vi "TempCtrlMonitor.vi"() -> ()   [LabVIEW 2015]
doc: "This is a control interface for using the digital temperature controller.\n\nThis interface is designed to be used in a stand-alone manner: a driver is also provided for low level, programmatic control and is used in the implementation of this GUI (see YbTempCtrl.lvlib)."
uses:
  Driver/Typedefs/OutputChannelTypedef.ctl
  Driver/Typedefs/InputChannelTypedef.ctl
  controls/ChannelSelection.ctl
  controls/ChannelSettings.ctl
  controls/UI Data.ctl
  controls/BridgeSettings.ctl
  <vilib>/Utility/error.llb/DialogType.ctl
  support/Message Queue/Enqueue Message (Single).vi
  support/Message Queue/Enqueue Message (Array).vi
  <vilib>/Utility/error.llb/Error Cluster From Error Code.vi
  <vilib>/ErrorRing/Error Ring.xnode
  support/Message Queue/Message Queue.lvlib
  support/User Event - Stop/User Event - Stop.lvlib
  Driver/YbTempCtrl.lvlib
panel:
  out "Data is logging":bool
  in  "Trigger time / s":i32=5 min=1
  in  "Tab Control":enum32{"Logging", "Control"}(tab)
  in  "Config input channel selector":T1
  in  "Input arm settings":T3(array[cluster])=[{"Enum string"="1T", "Enum ID"=0, "Input arm settings"={"Convert?"=FALSE, "Config"={"Vref"=1.25, "Rgain"=100000.0, "Rset"=10000.0, "Rseries"=1000.0, "Input polarity?"=FALSE}}}, {"Enum string"="2T", "Enum ID"=1, "Input arm settings"={"Convert?"=FALSE, "Config"={"Vref"=1.25, "Rgain"=100000.0, "Rset"=10000.0, "Rseries"=1000.0, "Input polarity?"=FALSE}}}, {"Enum string"="TMP", "Enum ID"=2, "Input arm settings"={"Convert?"=FALSE, "Config"={"Vref"=1.25, "Rgain"=100000.0, "Rset"=10000.0, "Rseries"=1000.0, "Input polarity?"=FALSE}}}, {"Enum string"="POW", "Enum ID"=3, "Input arm settings"={"Convert?"=FALSE, "Config"={"Vref"=1.25, "Rgain"=100000.0, "Rset"=10000.0, "Rseries"=1000.0, "Input polarity?"=FALSE}}}]
  in  "Output channel selection":T4=[{"Channel name"="1", "Enum id"=0, "Logging?"=FALSE}, {"Channel name"="2", "Enum id"=1, "Logging?"=FALSE}, {"Channel name"="3", "Enum id"=2, "Logging?"=FALSE}, {"Channel name"="4", "Enum id"=3, "Logging?"=FALSE}, {"Channel name"="BPA", "Enum id"=4, "Logging?"=FALSE}, {"Channel name"="BPB", "Enum id"=5, "Logging?"=FALSE}]
  in  "Input channel selection":T4=[{"Channel name"="1T", "Enum id"=0, "Logging?"=FALSE}, {"Channel name"="2T", "Enum id"=1, "Logging?"=FALSE}, {"Channel name"="TMP", "Enum id"=2, "Logging?"=FALSE}, {"Channel name"="POW", "Enum id"=3, "Logging?"=FALSE}]
  in  "Enable logging":bool
  in  "Log file prefix":string="Temperature log"
  in  "Log file directory":path
  in  "Reset":bool
  in  "VISA resource name":refnum<visa-resource-name>
  in  "Error alert group":enum32{"Page 1", "Page 2"}(tab)
  in  "Error abort":bool
  in  "Error ignore":bool
  out "Reported Error":string="20:32:20.341 21/11/2016 - Code -1073807346: 'VISA Open in YbTempCtrl.lvlib:Initialize.vi->TempCtrlMonitor.vi'"
  out "Output error":errorcluster={"status"=TRUE, "code"=-1073807346, "source"="VISA Write in YbTempCtrl.lvlib:Query-ControlSignal.vi->TempCtrlMonitor.vi"}
  out "Input error":errorcluster={"status"=TRUE, "code"=9999, "source"="Error from device: \"\""}
  out "Reading":dbl(graph)=nan
  in  "Input channel":T1
  in  "Output channel":T5
  in  "Start Lock":bool caption="Start Lock Outer"
  in  "Start Const.Voltage":bool caption="Start Lock Outer"
  in  "CtrlVoltage":dbl=nan caption="Output voltage / V"
  in  "Min_Ctrl":dbl caption="Minimum / V"
  in  "Max_Ctrl":dbl caption="Maximum / V"
  in  "Lock settings":T6={"K / V/V"=0.0, "T_I / s"=0.0, "T_D / s"=0.0, "Target Error / C"=0.0, "N"=10.0}
  in  "Exit":bool
  # "Log file setup"
  # "VISA config"
  # "Select which channels should be logged here. These will \nbe written to the log file regardless of which channel is \ndisplayed in the \"Control\" tab as long as \"Enable logging\" \nis set."
  # "Thermistor config"
  # "Enter the settings associated with a particular channel\nhere and then select \"Convert?\" in order to convert \nvoltages to temperatures on display\nN.B. Log files always contain raw voltages"
  # "Log files will be created with the current date and time appended to the prefix given here"
  # "Error reported:"
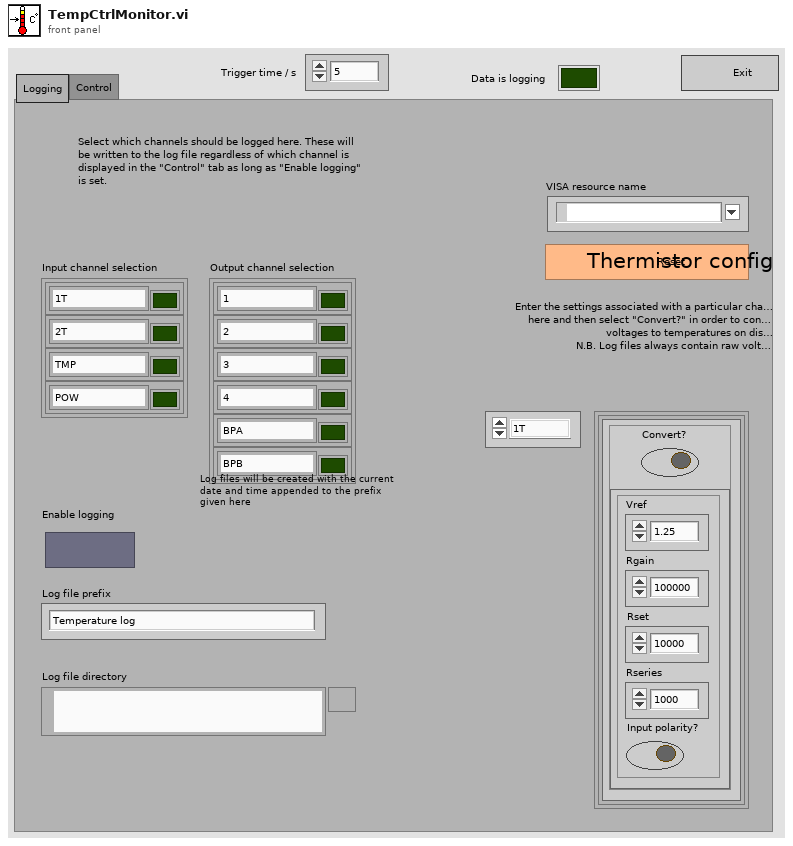
[diagram p1: front panel]
types:
  T1 = typedef "YbTempCtrl.lvlib/InputChannelTypedef.ctl" = enum16{"1T", "2T", "TMP", "POW"}
  T2 = typedef "ChannelSettings.ctl" = cluster{"Convert?":bool, "Config":cluster{"Vref":dbl, "Rgain":dbl, "Rset":dbl, "Rseries":dbl, "Input polarity?":bool}}
  T3 = cluster{"Enum string":string, "Enum ID":i16, "Input arm settings":T2}[]
  T4 = typedef "ChannelSelection.ctl" = cluster{"Channel name":string, "Enum id":u16, "Logging?":bool}[]
  T5 = typedef "YbTempCtrl.lvlib/OutputChannelTypedef.ctl" = enum16{"1", "2", "3", "4", "BPA", "BPB"}
  T6 = cluster{"K / V/V":dbl, "T_I / s":dbl, "T_D / s":dbl, "Target Error / C":dbl, "N":dbl}
  T7 = typedef "UI Data.ctl" = cluster{"VISA resource name":refnum<visa-resource-name>, "Log dir":refnum<vi>, "Log file":refnum<file>, "Outer PID State":string, "Inner PID State":string, "MAX_VOLTAGE":dbl, "Channel 1 bridge settings":T8, "Channel 2 bridge settings":T8, "Current Levels":cluster{"Control 1":dbl, "Control 2":dbl, "Control BP":dbl, "Error 1t":dbl, "Error 1v":dbl, "Error 2t":dbl, "Error 2v":dbl}, "Data is logging":refnum<vi>, "Output channel ref":refnum<vi>, "Output channel selection ref":refnum<vi>, "Input channel ref":refnum<vi>, "Input channel selection ref":refnum<vi>, "Log data?":bool, "Error reported?":bool, "Input arm settings":cluster{"Enum string":string, "Enum ID":i16, "Input arm settings":T2}[], "Input arm settings ref":refnum<vi>}
  T8 = typedef "BridgeSettings.ctl" = cluster{"Rgain":dbl, "Rset":dbl, "Vref":dbl, "Input polarity?":bool, "Rtherm_25":dbl}
  T9 = typedef "Message Queue.lvlib/All Message Queues.ctl" = cluster{"UI":refnum<queue>}
  T10 = enum8{"Enabled", "Disabled", "Disabled and Grayed Out"}
  T11 = typedef "YbTempCtrl.lvlib/OutputChannelTypedef.ctl" = enum16{"1", "2", "BP"}
  T12 = cluster{"K":dbl, "T_I / s":dbl, "T_D / s":dbl, "Target Error / V":dbl, "N":dbl}
  T13 = cluster{"Lock settings":cluster{"K":dbl, "T_I / s":dbl, "T_D / s":dbl, "Target Error / C":dbl, "N":dbl}, "Output channel":T5, "Input channel":T1}
  T14 = cluster{"Output channel":T5, "Max_Ctrl1":dbl, "Min_Ctrl1":dbl}
  T15 = cluster{"Output channel":T5, "Voltage outer":dbl}
  T16 = typedef "DialogType.ctl" = u16
  T17 = cluster{"seconds since 1Jan1904":timestamp, dbl[]}
  T18 = cluster{"K":dbl, "T_I / s":dbl, "T_D / s":dbl, "Target Error / C":dbl, "N":dbl}
  T19 = cluster{"Enum string":string, "Enum ID":i16, "Input arm settings":T2}
  T20 = cluster{"Vref":dbl, "Rgain":dbl, "Rset":dbl, "Rseries":dbl, "Input polarity?":bool}
  T21 = cluster{"Lock settings":cluster{"K / V/V":dbl, "T_I / s":dbl, "T_D / s":dbl, "Target Error / C":dbl, "N":dbl}, "Output channel":T5, "Input channel":T1}
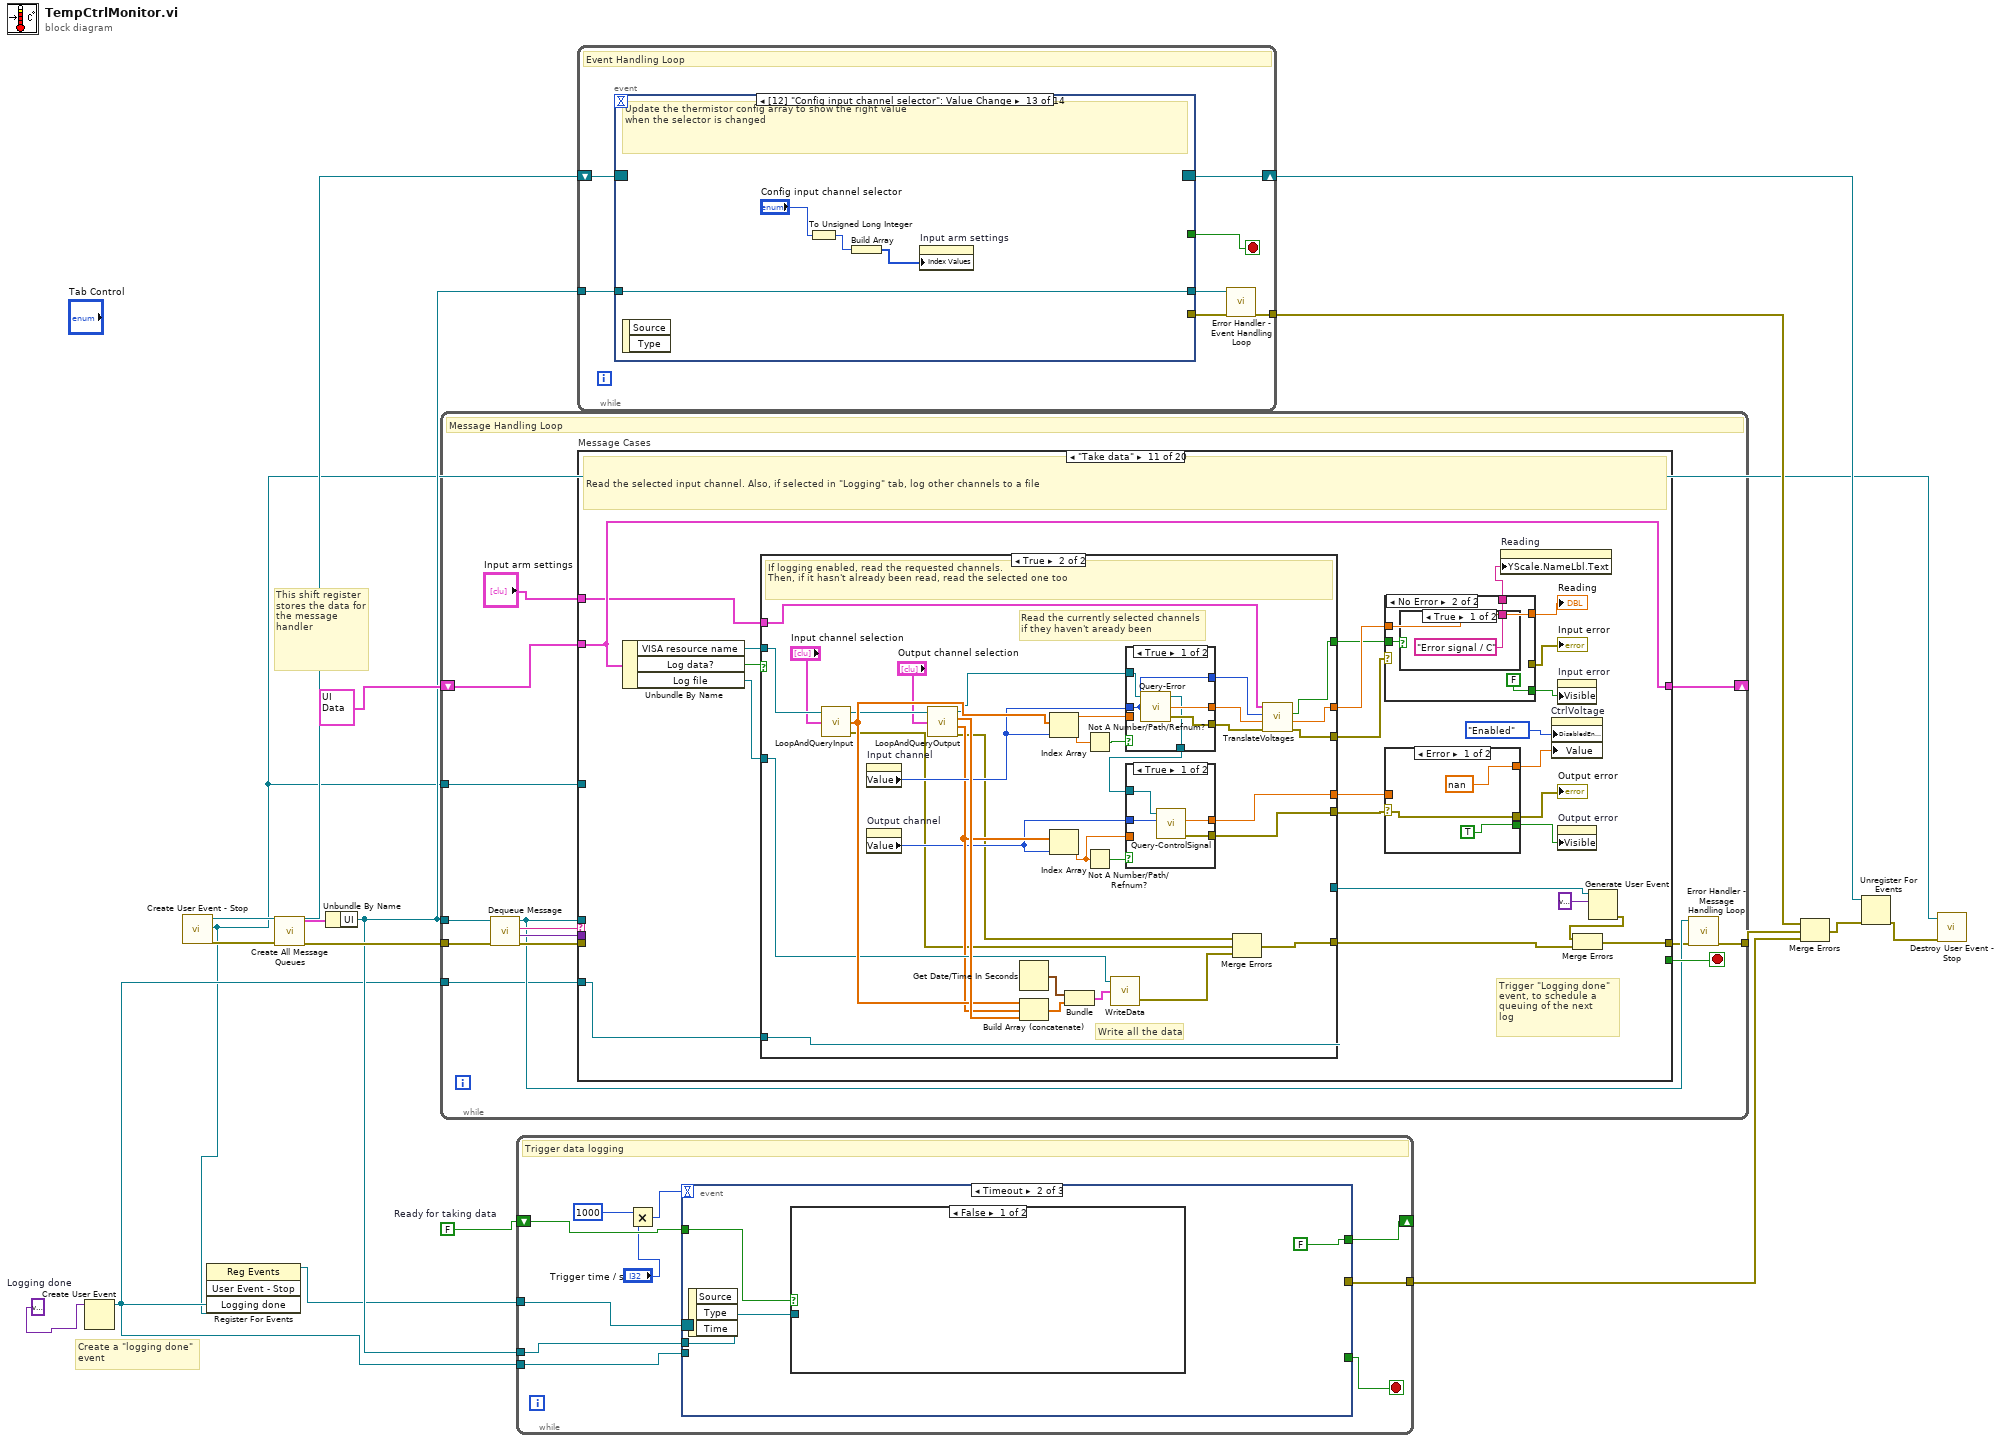
[diagram p0: block diagram]
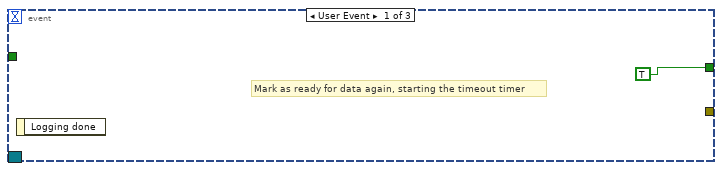
[diagram p2: hidden frame]
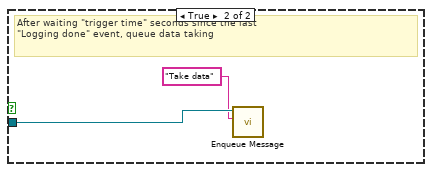
[diagram p3: hidden frame]
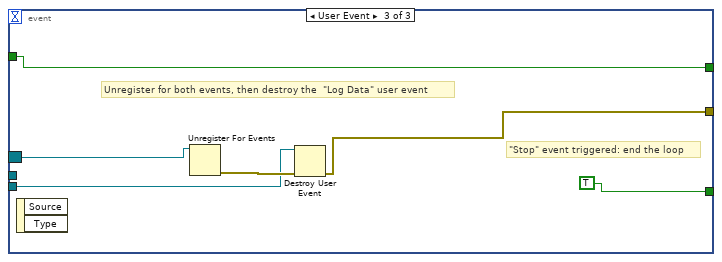
[diagram p4: hidden frame]
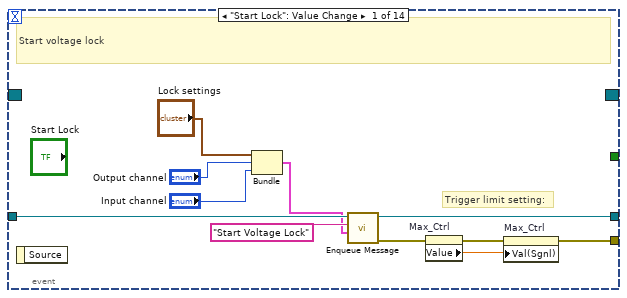
[diagram p5: hidden frame]
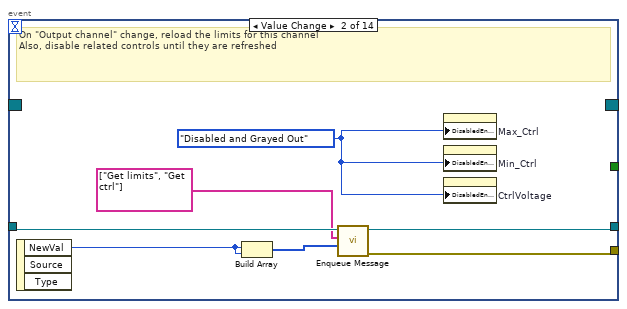
[diagram p6: hidden frame]
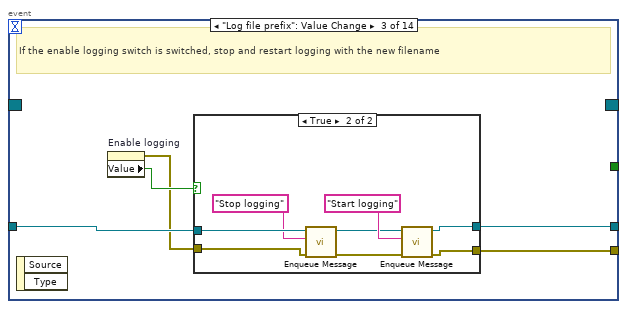
[diagram p7: hidden frame]
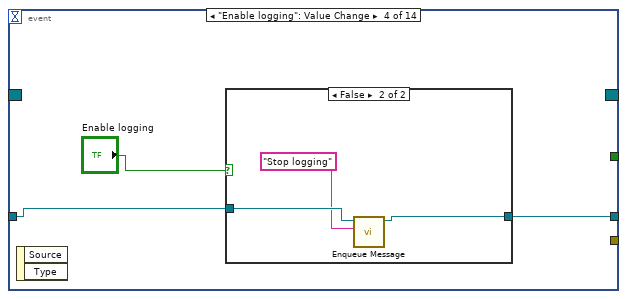
[diagram p9: hidden frame]
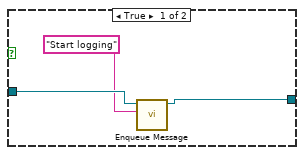
[diagram p10: hidden frame]
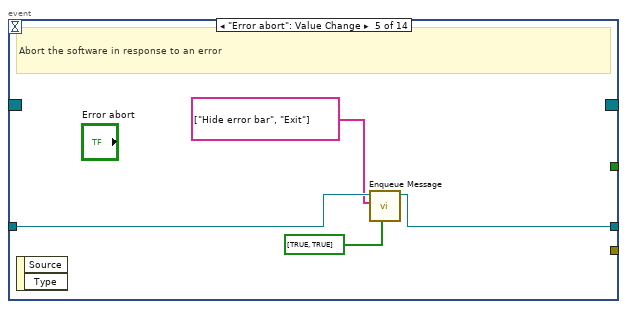
[diagram p11: hidden frame]
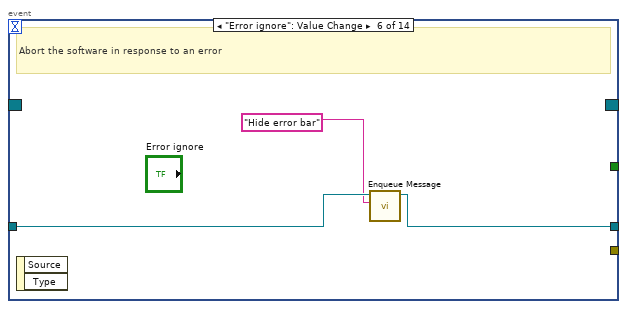
[diagram p12: hidden frame]
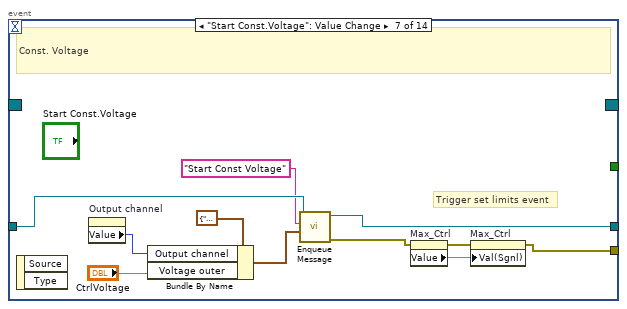
[diagram p13: hidden frame]
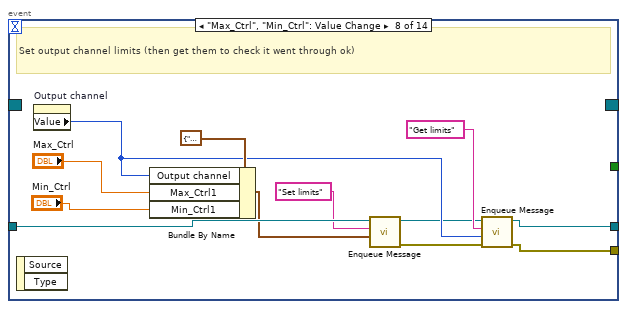
[diagram p14: hidden frame]
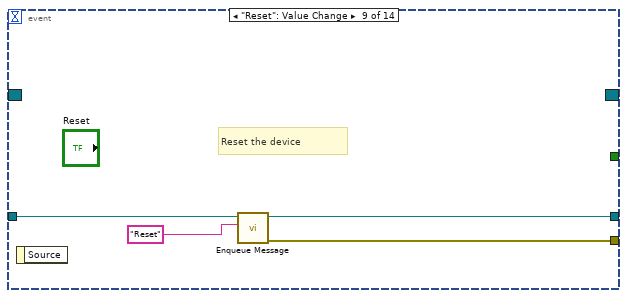
[diagram p15: hidden frame]
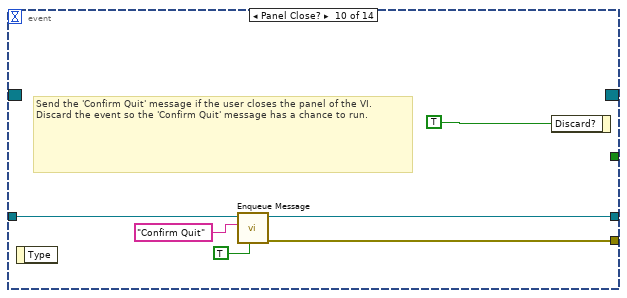
[diagram p16: hidden frame]
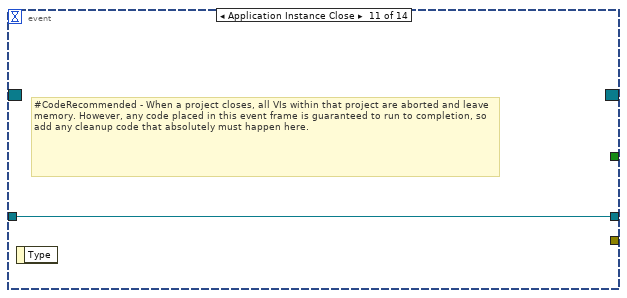
[diagram p17: hidden frame]
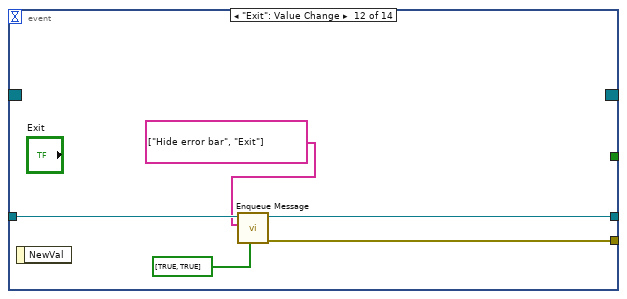
[diagram p18: hidden frame]
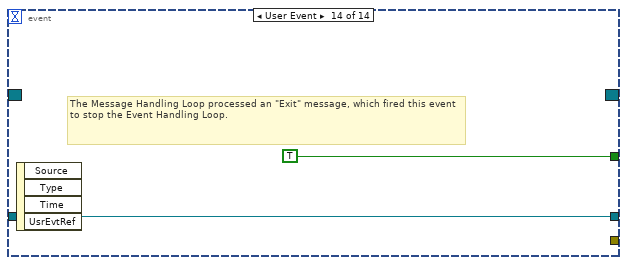
[diagram p19: hidden frame]
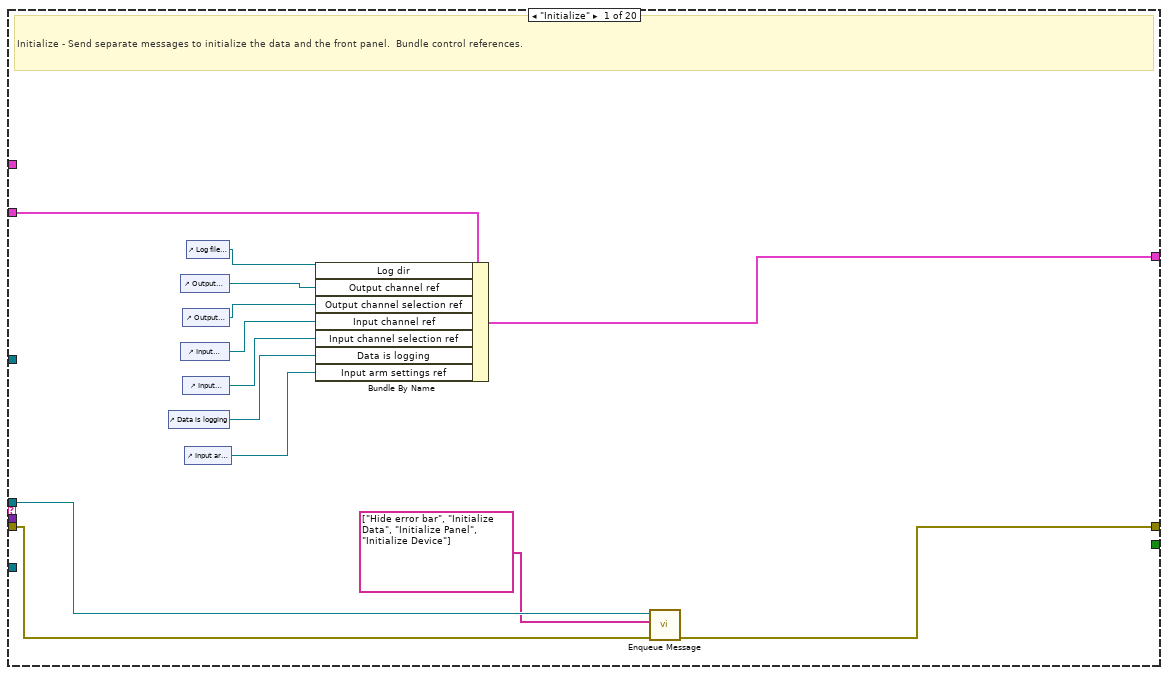
[diagram p20: hidden frame]
diagram:
  w1 = FALSE  # Ready for taking data
  w8 = variant  # Logging done
  # "Create a \"logging done\"\nevent"
  # "This shift register stores the data for the message handler"
  n1 = Create User Event(user event datatype=w8) -> (user event=w4:refnum<user-event>)  [unwired: 1 in, 1 out]
  n2 = call "Create User Event - Stop.vi"() -> ("error out"=w15:errorcluster, "User Event - Stop"=w3:refnum<user-event>, "Stop Event Registration Refnum"=w9:refnum<event-registration>)  [unwired: 9 in]
  n3 = register-events(w3, w4) -> (reference out=w2:refnum<event-registration>)  [unwired: 2 in, 1 out]
  n4 = call "Create All Message Queues.vi"("error in (no error)"=w15) -> ("error out"=w17:errorcluster, "Message Queues out"=w16:T9)  [unwired: 9 in]
  n5 = Unbundle By Name(w16) -> ("UI"=w10:refnum<queue>)
  n6 = while {
    tunnel: w10 -> [w23]
    shift-right: [w30] -> _
    shift-left: T7 {"VISA resource name"="", "Log dir"=refnum, "Log file"=refnum, "Outer PID State"="", "Inner PID State"="", "MAX_VOLTAGE"=0.0, "Channel 1 bridge settings"={"Rgain"=0.0, "Rset"=0.0, "Vref"=0.0, "Input polarity?"=FALSE, "Rtherm_25"=0.0}, "Channel 2 bridge settings"={"Rgain"=0.0, "Rset"=0.0, "Vref"=0.0, "Input polarity?"=FALSE, "Rtherm_25"=0.0}, "Current Levels"={"Control 1"=0.0, "Control 2"=0.0, "Control BP"=0.0, "Error 1t"=0.0, "Error 1v"=0.0, "Error 2t"=0.0, "Error 2v"=0.0}, "Data is logging"=refnum, "Output channel ref"=refnum, "Output channel selection ref"=refnum, "Input channel ref"=refnum, "Input channel selection ref"=refnum, "Log data?"=FALSE, "Error reported?"=FALSE, "Input arm settings"=[], "Input arm settings ref"=refnum} ("Data Cluster") -> [w31]
    tunnel: w3 -> [w28]
    tunnel: w17 -> [w27]
    tunnel: [w21] -> w7
    tunnel: w4 -> [w19]
    stop <- w29 stop-if-true
    # "Message Handling Loop"
    n7 = call "Dequeue Message.vi"("error in (no error)"=w27, "Message Queue"=w23) -> ("error out"=w26:errorcluster, "Message Data"=w24:variant, "Message"=w25:string, "dup Message Queue"=w22:refnum<queue>)  [unwired: 6 in]
    n8 = case "Message Cases" shown="\"Take data\"" w25 {
      selector: w25 -> [_ _ _ _ _ _ _ _ _ _ _ _ _ _ _ _ _ _ _ w399]
      tunnel: w22 -> [w42 _ w58 w89 _ w143 _ _ _ w174 _ _ w324 w337 _ _ _ _ w398 _]
      tunnel: w26 -> [w43 w55 w60 _ w121 w147 w150 w155 w164 w177 _ w286 w325 w339 _ _ _ _ w395 _]
      tunnel: [w44 w52 w63 w108 w119 w145 w148 w154 w165 w173 w204 w289 w322 w341 w342 w356 w374 w386 w396 w400] -> w20
      tunnel: w31 -> [w41 w54 w62 w104 w117 w146 w149 w153 w159 w170 w187 w288 w302 w340 w348 w364 w376 w384 w393 w401]
      tunnel: [w40 w53 w62 w103 w116 w146 w149 w152 w158 w179 w187 w288 w302 w340 w348 w364 w376 w384 w393 w401] -> w30
      tunnel: [_ _ _ _ _ _ _ _ _ _ _ _ _ _ _ _ _ _ TRUE _] -> w29
      tunnel: w24 -> [_ _ _ _ w120 _ _ _ _ _ _ _ w327 _ w349 w365 w377 w385 _ _]
      tunnel: w28 -> [_ _ _ _ _ _ _ _ _ _ _ _ _ _ _ _ _ _ w394 _]
      tunnel: w19 -> [_ _ _ _ _ _ _ _ _ _ w207 _ _ _ _ _ _ _ _ _]
      tunnel: "Input arm settings" -> [_ _ _ _ _ _ _ _ _ _ w186 _ w308 _ _ _ _ _ _ _]
      frame "Initialize" {
        # "Initialize - Send separate messages to initialize the data and the front panel.  Bundle control references."
        n9 = control-ref of="Data is logging"() -> (w33:refnum<vi>)
        n10 = control-ref of="Output channel"() -> (w37:refnum<vi>)
        n11 = control-ref of="Input channel"() -> (w36:refnum<vi>)
        n12 = control-ref of="Output channel selection"() -> (w34:refnum<vi>)
        n13 = control-ref of="Input channel selection"() -> (w35:refnum<vi>)
        n14 = control-ref of="Input arm settings"() -> (w32:refnum<vi>)
        n15 = control-ref of="Log file directory"() -> (w39:refnum<vi>)
        n16 = Bundle By Name(cluster=w41, "Log dir"=w39, "Output channel ref"=w37, "Output channel selection ref"=w34, "Input channel ref"=w36, "Input channel selection ref"=w35, "Data is logging"=w33, "Input arm settings ref"=w32) -> (w40:T7)
        n17 = call-poly "Enqueue Message.vi"("error in (no error)"=w43, "Message Array"=string[] ["Hide error bar", "Initialize Data", "Initialize Panel", "Initialize Device"], "Message Queue"=w42) -> ("error out"=w44:errorcluster)  [unwired: 7 in, 1 out]
      }
      frame "Initialize Data" {
        w45 = nan
        w51 = "?"
        # "Initialize Data - Initialize the state data cluster."
        n18 = Bundle(w45, w45, w45, w45, w45, w45, w45) -> (w46:cluster{dbl, dbl, dbl, dbl, dbl, dbl, dbl})  [unwired: 1 in]
        n19 = Bundle By Name(cluster=w54, "VISA resource name"="VISA resource name", "Outer PID State"=w51, "Inner PID State"=w51, "MAX_VOLTAGE"=15.0, "Channel 1 bridge settings"=T8 {"Rgain"=42000.0, "Rset"=9500.0, "Vref"=1.0, "Input polarity?"=FALSE, "Rtherm_25"=10000.0}, "Channel 2 bridge settings"=T8 {"Rgain"=42000.0, "Rset"=9500.0, "Vref"=1.0, "Input polarity?"=FALSE, "Rtherm_25"=10000.0} ("Channel 1 bridge settings"), "Current Levels"=w46) -> (w53:T7)
        n20 = Merge Errors(w55) -> (w52:errorcluster)
      }
      frame "Initialize Device" {
        # "No reset"
        # "Initialize Device - Start comms with the PID controller"
        n21 = Unbundle By Name(w62) -> ("VISA resource name"=w56:refnum<visa-resource-name>)
        n22 = call "Initialize.vi"("error in (no error)"=w60, "Reset (True)"=FALSE, "VISA resource name"=w56) -> ("error out"=w59:errorcluster)  [unwired: 7 in, 1 out]
        n23 = case shown="Error" w59 {
          selector: w59 -> [w64 w76]
          tunnel: w58 -> [_ w72]
          tunnel: [w64 w69] -> w57
          tunnel: w56 -> [_ w65]
          frame No Error {
            # "No error"
          }
          frame Error {
            w75 = T16 0 items=["no dialog", "OK message", "continue or stop message", "OK message + warnings", "continue/stop + warnings"] ("type of dialog (OK msg:1)")
            # "Error initialising the device. Abort execution since there's\nno point continuing. (This code is here to override the default\nerror handler which would just pop up an error bar)"
            n24 = call <vilib>:"Simple Error Handler.vi"("type of dialog (OK msg:1)"=w75, "error in (no error)"=w76) -> ("code out"=w66:i32, "source out"=w67:string)  [unwired: 3 in, 3 out]
            n25 = Format Into String(format string="An error occured in device initialisation.\nCOM port: \"%s\"\nError code: %d\nError message: \"%s\"", w65, w66, w67) -> (resulting string=w73:string)  [unwired: 2 in, 1 out]
            n26 = One Button Dialog(message=w73, button name ("OK")="Abort...") -> ()  [unwired: 1 out]
            n27 = call-poly "Enqueue Message.vi"("Priority Message? (F)"=TRUE, "Message"="Exit", "Message Queue"=w72) -> ("error out"=w69:errorcluster)  [unwired: 7 in, 1 out]
          }
        }
        n28 = Merge Errors(w57) -> (w63:errorcluster)
      }
      frame "Initialize Panel" {
        w95 = FALSE
        # "Trigger the index changed event"
        # "Trigger taking of first data\nFrom here on, \"Take data\" will retrigger itself"
        # "Trigger reloading of limits"
        # "Set logging indicators to false (they will be updated later)"
        # "Initialize Panel - Initialize the appearance of the front panel here."
        n29 = Unbundle By Name(w104) -> ("Data is logging"=w107:refnum<vi>, "Output channel ref"=w106:refnum<vi>, "Output channel selection ref"=w105:refnum<vi>, "Input channel ref"=w102:refnum<vi>, "Input channel selection ref"=w101:refnum<vi>, "Input channel ref"=w88:refnum<vi>, "Input arm settings ref"=w82:refnum<vi>)
        n30 = property on="Output channel" class="Enum (strict)"() -> ("Value"=w99:T5)  [unwired: 2 in, 2 out]
        n31 = call-poly "Enqueue Message.vi"("Message Data"=w99, "Message"="Get limits", "Message Queue"=w89) -> ("error out"=w94:errorcluster, "dup Message Queue"=w93:refnum<queue>)  [unwired: 7 in]
        n32 = property on="Enable logging" class="Bool (strict)"() -> ("Value"=w96:bool)  [unwired: 2 in, 2 out]
        n33 = property class="Bool (strict)"(reference=w107, "Value"=w95) -> (error out=w86:errorcluster)  [unwired: 1 in, 1 out]
        n34 = Bundle By Name(cluster=w104, "Log data?"=w95) -> (w103:T7)
        n35 = case shown="True" w96 {
          tunnel: w94 -> [w110 w115]
          tunnel: w93 -> [w109 w114]
          tunnel: "Start logging" ("Message") -> [_ w113]
          tunnel: [w110 w112] -> w91
          tunnel: [w109 w111] -> w90
          frame False {
          }
          frame True {
            n36 = call-poly "Enqueue Message.vi"("error in (no error)"=w115, "Message"=w113, "Message Queue"=w114) -> ("error out"=w112:errorcluster, "dup Message Queue"=w111:refnum<queue>)  [unwired: 7 in]
          }
        }
        n37 = control-ref of="Config input channel selector"() -> (w77:refnum<vi>)
        n38 = call "PopulateChannelArray.vi"("Channel Selection ref"=w105, "Enum in"=w106) -> ("error out"=w85:errorcluster)  [unwired: 2 in]
        n39 = call "PopulateChannelArray.vi"("Channel Selection ref"=w101, "Enum in"=w102) -> ("error out"=w84:errorcluster)  [unwired: 2 in]
        n40 = call "PopulateChannelSettingsArray.vi"("Update size?"=FALSE, "Input arm settings ref"=w82, "Enum in"=w88) -> ("error out"=w81:errorcluster)  [unwired: 1 in]
        n41 = property class="Enum (strict)"(reference=w77, error in=w81) -> (reference out=w78:refnum<vi>, error out=w79:errorcluster, "Value"=w80:T1)
        n42 = call-poly "Enqueue Message.vi"("error in (no error)"=w91, "Message"="Take data", "Message Queue"=w90) -> ("error out"=w92:errorcluster)  [unwired: 7 in, 1 out]
        n43 = property class="Enum (strict)"(reference=w78, error in=w79, "Val(Sgnl)"=w80) -> (error out=w83:errorcluster)  [unwired: 1 out]
        n44 = Merge Errors(w86, w85, w84, w83, w92) -> (w108:errorcluster)
      }
      frame "Error" {
        # "#CodeRecommended - If you ever change the name of this \"Error\" message, you'll need to update the name in the Check Loop Error.vi as well."
        # "Error - Check the error message data and respond accordingly. This message is sent by the \"Error Handler\" VIs at the end of each loop in this application.\n\nResponse: show the error alert box, allowing the user to abort the program"
        n45 = Unbundle By Name(w117) -> ("Error reported?"=w118:bool)
        n46 = case shown="False" w118 {
          tunnel: w121 -> [w138 w140]
          tunnel: w120 -> [w137 _]
          tunnel: [w128 w140] -> w119
          tunnel: w117 -> [w124 w139]
          tunnel: [w123 w139] -> w116
          frame False {
            w134 = T16 0 items=["no dialog", "OK message", "continue or stop message", "OK message + warnings", "continue/stop + warnings"] ("type of dialog (OK msg:1)")
            # "Show the error bar"
            # "The error bar is not yet visible. Populate it with details of the error then show it"
            n47 = Variant To Data(error in=w138, type=errorcluster {"status"=FALSE, "code"=0, "source"=""} ("error constant"), Variant=w137) -> (data=w135:errorcluster, error out=w131:errorcluster)
            n48 = Get Date/Time In Seconds() -> (seconds since 1Jan1904=w125:timestamp)
            n49 = call <vilib>:"Simple Error Handler.vi"("type of dialog (OK msg:1)"=w134, "error in (no error)"=w135) -> ("code out"=w126:i32, "source out"=w127:string)  [unwired: 3 in, 3 out]
            n50 = Format Into String(format string="%T - Code %d: '%s'", error in=w131, w125, w126, w127) -> (resulting string=→"Reported Error":string, error out=w129:errorcluster)  [unwired: 1 in]
            n51 = Bundle By Name(cluster=w124, "Error reported?"=TRUE) -> (w123:T7)
            n52 = property on="Error alert group" class="TabCtl (strict)"(error in=w129, "Visible"=TRUE) -> (error out=w128:errorcluster)  [unwired: 1 in, 1 out]
          }
          frame True {
            # "An error is already visible. Leave it, since it's probably more useful than newer errors"
          }
        }
      }
      frame "Confirm Quit" {
        # "#CodeNeeded - If you want to provide an \"Are you sure\" dialog (or some other notification) before the application exits, place that code here. This message is typically sent from a Panel Close? event."
        # "Confirm Quit - Message that can confirm whether or not the user wants to exit the application."
        n53 = call-poly "Enqueue Message.vi"("Priority Message? (F)"=TRUE, "error in (no error)"=w147, "Message"="Exit", "Message Queue"=w143) -> ("error out"=w144:errorcluster)  [unwired: 6 in, 1 out]
        n54 = Merge Errors(w144) -> (w145:errorcluster)
      }
      frame "---Copy This Frame---" {
        # "Duplicate this frame when creating new messages.  Change this comment in the duplicated frame to describe this message."
        n55 = Merge Errors(w150) -> (w148:errorcluster)
      }
      frame "Hide error bar" {
        # "Hide the error bar"
        n56 = Bundle By Name(cluster=w153, "Error reported?"=FALSE) -> (w152:T7)
        n57 = property on="Error alert group" class="TabCtl (strict)"(error in=w155, "Visible"=FALSE) -> (error out=w154:errorcluster)  [unwired: 1 in, 1 out]
      }
      frame "Stop logging" {
        # "Mark logging as disabed: the event will not get re-triggered so logging will stop"
        n58 = Unbundle By Name(w159) -> ("Log file"=w162:refnum<file>)
        n59 = Not A Number/Path/Refnum?(number/path/refnum=w162) -> (NaN/Path/Refnum?=w161:bool)
        n60 = case shown="False" w161 {
          tunnel: w164 -> [w168 w169]
          tunnel: [w167 w169] -> w163
          tunnel: w162 -> [w166 _]
          frame False {
            n61 = Close File(refnum=w166, error in=w168) -> (error out=w167:errorcluster)  [unwired: 1 out]
          }
          frame True {
          }
        }
        n62 = Bundle By Name(cluster=w159, "Log data?"=FALSE, "Log file"=refnum<k0> refnum) -> (w158:T7)
        n63 = Merge Errors(w163) -> (w165:errorcluster)
      }
      frame "Start logging" {
        # "Open files for data logging with the given headers"
        n64 = call "GenFilenames.vi"("Controller name"="Log file prefix", "Default dir"="Log file directory") -> ("Log file"=w180:path)  [unwired: 1 in]
        n65 = call "GenerateHeaders.vi"("UI Data"=w170) -> ("Output headers"=w171:string)  [unwired: 1 in]
        n66 = call "OpenFile.vi"("error in (no error)"=w177, "Filepath"=w180, "Extra headers"=w171) -> ("error out"=w176:errorcluster, "File handle"=w178:refnum<file>)
        n67 = case shown="Error" w176 {
          selector: w176 -> [w182 w184]
          tunnel: [TRUE ("Data is logging") FALSE ("Data is logging")] -> w172
          tunnel: w174 -> [_ _]
          tunnel: [w182 _] -> w173
          frame No Error {
            # "Mark logging as enabled"
          }
          frame Error {
            # "Opening files failed! Report error"
            n68 = call <vilib>:"Simple Error Handler.vi"("error in (no error)"=w184) -> ()  [unwired: 4 in, 5 out]
          }
        }
        "Data is logging" <- w172
        n69 = Bundle By Name(cluster=w170, "Log file"=w178, "Log data?"=w172) -> (w179:T7)
        n70 = property on="Enable logging" class="Bool (strict)"("Value"=w172) -> ()  [unwired: 2 in, 2 out]
      }
      frame "Take data" {
        # "Trigger \"Logging done\"\nevent, to schedule a\nqueuing of the next\nlog"
        # "Read the selected input channel. Also, if selected in \"Logging\" tab, log other channels to a file"
        n71 = Unbundle By Name(w187) -> ("VISA resource name"=w209:refnum<visa-resource-name>, "Log data?"=w208:bool, "Log file"=w200:refnum<file>)
        n72 = case shown="True" w208 {
          tunnel: w209 -> [w237 w271]
          tunnel: [_ w266] -> w202
          tunnel: w207 -> [w238 w261]
          tunnel: [w228 w243] -> w196
          tunnel: [w238 w261] -> w205
          tunnel: [w232 w244] -> w201
          tunnel: w200 -> [_ w257]
          tunnel: [w234 w248] -> w193
          tunnel: [w233 w252] -> w192
          tunnel: [w227 w242] -> w191
          tunnel: w186 -> [w226 w241]
          frame False {
            # "If logging disabled, just read the currently selected channels"
            n73 = property on="Input channel" class="Enum (strict)"() -> ("Value"=w229:T1)  [unwired: 2 in, 2 out]
            n74 = property on="Output channel" class="Enum (strict)"() -> ("Value"=w236:T5)  [unwired: 2 in, 2 out]
            n75 = call "Query-Error.vi"("Input channel"=w229, "VISA resource name"=w237) -> ("error out"=w231:errorcluster, "Error Signal / V"=w230:dbl, "VISA resource name out"=w235:refnum<visa-resource-name>)  [unwired: 1 in]
            n76 = call "Query-ControlSignal.vi"("Output channel"=w236, "VISA resource name"=w235) -> ("error out"=w234:errorcluster, "Recalled Control signal / V"=w233:dbl)  [unwired: 7 in, 1 out]
            n77 = call "TranslateVoltages.vi"("Input arm settings"=w226, "Input channel"=w229, "Reading / V"=w230, "error in (no error)"=w231) -> ("Output is temperature?"=w227:bool, "Output"=w228:dbl, "error out"=w232:errorcluster)  [unwired: 1 in, 2 out]
          }
          frame True {
            # "Read the currently selected channels\nif they haven't aready been"
            # "Write all the data"
            # "If logging enabled, read the requested channels. \nThen, if it hasn't already been read, read the selected one too"
            n78 = call "LoopAndQueryInput.vi"("Input channel selection"="Input channel selection", "VISA Refnum in"=w271) -> ("error out"=w239:errorcluster, "Error signal / V"=w265:dbl[], "VISA resource name out"=w260:refnum<visa-resource-name>)  [unwired: 1 in]
            n79 = property on="Input channel" class="Enum (strict)"() -> ("Value"=w263:T1)  [unwired: 2 in, 2 out]
            n80 = property on="Output channel" class="Enum (strict)"() -> ("Value"=w250:T5)  [unwired: 2 in, 2 out]
            n81 = call "LoopAndQueryOutput.vi"("VISA Refnum in"=w260, "Output channel selection"="Output channel selection") -> ("VISA resource name out"=w256:refnum<visa-resource-name>, "Setpoint / V"=w270:dbl[], "Control signal / V"=w253:dbl[], "error out"=w240:errorcluster)  [unwired: 1 in]
            n82 = Get Date/Time In Seconds() -> (seconds since 1Jan1904=w269:timestamp)
            n83 = Build Array (concatenate)(w265, w253, w270) -> (w268:dbl[])
            n84 = Index Array(array=w265, index=w263) -> (element=w262:dbl)
            n85 = Index Array(array=w253, index=w250) -> (element=w249:dbl)
            n86 = Bundle("seconds since 1Jan1904"=w269, w268) -> (w267:T17)  [unwired: 1 in]
            n87 = Not A Number/Path/Refnum?(number/path/refnum=w262) -> (NaN/Path/Refnum?=w264:bool)
            n88 = Not A Number/Path/Refnum?(number/path/refnum=w249) -> (NaN/Path/Refnum?=w254:bool)
            n89 = call "WriteData.vi"("Log data"=w267, "File handle"=w257) -> ("error out"=w255:errorcluster)  [unwired: 1 in, 1 out]
            n90 = case shown="True" w264 {
              tunnel: w263 -> [w277 w282]
              tunnel: [w281 w284] -> w246
              tunnel: w262 -> [_ w284]
              tunnel: [w280 _] -> w245
              tunnel: w256 -> [w279 w283]
              tunnel: [w278 w283] -> w251
              tunnel: [w277 w282] -> w247
              frame True {
                n91 = call "Query-Error.vi"("Input channel"=w277, "VISA resource name"=w279) -> ("error out"=w280:errorcluster, "Error Signal / V"=w281:dbl, "VISA resource name out"=w278:refnum<visa-resource-name>)  [unwired: 1 in]
              }
              frame False {
              }
            }
            n92 = case shown="True" w254 {
              tunnel: [w275 w276] -> w252
              tunnel: w251 -> [w274 _]
              tunnel: [w273 _] -> w248
              tunnel: w250 -> [w272 _]
              tunnel: w249 -> [_ w276]
              frame True {
                n93 = call "Query-ControlSignal.vi"("Output channel"=w272, "VISA resource name"=w274) -> ("error out"=w273:errorcluster, "Recalled Control signal / V"=w275:dbl)  [unwired: 7 in, 1 out]
              }
              frame False {
              }
            }
            n94 = Merge Errors(w240, w239, w255) -> (w266:errorcluster)
            n95 = call "TranslateVoltages.vi"("Input arm settings"=w241, "Input channel"=w247, "Reading / V"=w246, "error in (no error)"=w245) -> ("Output is temperature?"=w242:bool, "Output"=w243:dbl, "error out"=w244:errorcluster)  [unwired: 1 in, 2 out]
          }
        }
        n96 = case shown="No Error" w201 {
          selector: w201 -> [w219 _]
          tunnel: [w219 _] -> w199
          tunnel: [TRUE FALSE] -> w198
          tunnel: [nan ("Error Signal / V") w222] -> w197
          tunnel: w196 -> [_ w222]
          tunnel: w191 -> [_ w221]
          tunnel: ["" w220] -> w188
          frame Error {
          }
          frame No Error {
            n97 = case shown="True" w221 {
              tunnel: ["Error signal / C" "Error signal / V"] -> w220
              frame True {
              }
              frame False {
              }
            }
          }
        }
        "Reading" <- w197
        "Input error" <- w199
        n98 = case shown="Error" w193 {
          selector: w193 -> [w212 w215]
          tunnel: [w212 w215] -> w195
          tunnel: [TRUE FALSE] -> w194
          tunnel: [nan ("Error Signal / V") w213] -> w190
          tunnel: w192 -> [_ w213]
          frame Error {
          }
          frame No Error {
          }
        }
        "Output error" <- w195
        n99 = property on="Reading" class="WFChart (strict)"("YScale.NameLbl.Text"=w188) -> ()  [unwired: 2 in, 2 out]
        n100 = property on="CtrlVoltage" class="DigNum (strict)"("DisabledEnum"=T10."Enabled" ("Disabled"), "Value"=w190) -> ()  [unwired: 2 in, 2 out]
        n101 = property on="Input error" class="Clust (strict)"("Visible"=w198) -> ()  [unwired: 2 in, 2 out]
        n102 = property on="Output error" class="Clust (strict)"("Visible"=w194) -> ()  [unwired: 2 in, 2 out]
        n103 = Generate User Event(user event=w205, event data cluster=variant ("event data")) -> (error out=w203:errorcluster)  [unwired: 2 in, 1 out]
        n104 = Merge Errors(w203, w202) -> (w204:errorcluster)
      }
      frame "Check State" {
        # "Get the current status of the device"
        n105 = Unbundle By Name(w288) -> ("VISA resource name"=w287:refnum<visa-resource-name>)
        n106 = disable-structure shown="Disabled" {
          disable-tunnel: w287 -> [w299 _]
          disable-tunnel: w286 -> [w296 w300]
          disable-tunnel: [w293 w300] -> w285
          frame Disabled {
            n107 = call "Status.vi"("error in (no error)"=w296, "Output channel"=OutputChannelTypedef."1", "VISA resource name"=w299) -> ("error out"=w295:errorcluster, "VISA resource name out"=w298:refnum<visa-resource-name>)  [unwired: 1 out]
            n108 = call "Status.vi"("error in (no error)"=w295, "Output channel"=OutputChannelTypedef."2", "VISA resource name"=w298) -> ("error out"=w294:errorcluster, "VISA resource name out"=w297:refnum<visa-resource-name>)  [unwired: 1 out]
            n109 = call "Status.vi"("error in (no error)"=w294, "Output channel"=OutputChannelTypedef."BP", "VISA resource name"=w297) -> ("error out"=w293:errorcluster)  [unwired: 2 out]
          }
          frame Enabled {
          }
        }
        n110 = Merge Errors(w285) -> (w289:errorcluster)
      }
      frame "Start Voltage Lock" {
        # "Start lock with the given controller and given settings\nN.B. The event data variant must be a cluster, elements:\n0 - Cluster of PID settings\n1 - Required controller"
        n111 = Variant To Data(error in=w325, type=T13 {"Lock settings"={"K"=0.0, "T_I / s"=0.0, "T_D / s"=0.0, "Target Error / C"=0.0, "N"=0.0}, "Output channel"=enum."1", "Input channel"=enum."1T"} ("output cluster"), Variant=w327) -> (data=w326:T13, error out=w312:errorcluster)
        n112 = Unbundle By Name(w302) -> ("VISA resource name"=w316:refnum<visa-resource-name>)
        n113 = Unbundle By Name(w326) -> ("Lock settings"=w321:T18, "Input channel"=w307:T1, "Output channel"=w310:T5)
        n114 = Index Array(array=w308, index=w307) -> (element=w306:T19)
        n115 = Unbundle By Name(w321) -> ("Target Error / C"=w309:dbl, "K"=w320:dbl, "T_I / s"=w319:dbl, "T_D / s"=w318:dbl, "N"=w317:dbl)
        n116 = Unbundle By Name(w306) -> ("Input arm settings"=w305:T2)
        n117 = Unbundle By Name(w305) -> ("Config"=w304:T20)
        n118 = call "ConvertToADCReading.vi"("Temperature / C"=w309, "Input arm settings"=w304) -> ("Reading / V"=w303:dbl)  [unwired: 1 out]
        n119 = Bundle By Name(cluster=T12 {"K"=0.0, "T_I / s"=0.0, "T_D / s"=0.0, "Target Error / V"=0.0, "N"=10.0} ("Lock settings"), "Target Error / V"=w303, "K"=w320, "T_I / s"=w319, "T_D / s"=w318, "N"=w317) -> (w313:T12)
        n120 = call "StartLock.vi"("VISA resource name"=w316, "Input channel"=w307, "Output channel"=w310, "Lock settings"=w313, "error in (no error)"=w312) -> ("error out"=w311:errorcluster)  [unwired: 8 in, 2 out]
        n121 = Unbundle By Name(w302) -> ("Log data?"=w301:bool)
        n122 = case shown="True" w301 {
          tunnel: w324 -> [_ w332]
          tunnel: [w328 w331] -> w323
          tunnel: w311 -> [w328 w330]
          frame False {
            # "No logging: do nothing"
          }
          frame True {
            # "Logging data on: restart"
            n123 = call-poly "Enqueue Message.vi"("error in (no error)"=w330, "Message Array"=string[] ["Stop logging", "Start logging"], "Message Queue"=w332) -> ("error out"=w331:errorcluster)  [unwired: 7 in, 1 out]
          }
        }
        n124 = Merge Errors(w323) -> (w322:errorcluster)
      }
      frame "Reset" {
        # "High priority"
        # "Reinitialize"
        # "Reset the device"
        n125 = Unbundle By Name(w340) -> ("VISA resource name"=w338:refnum<visa-resource-name>)
        n126 = call "Reset.vi"("error in (no error)"=w339, "VISA resource name"=w338) -> ("error out"=w336:errorcluster)  [unwired: 8 in, 1 out]
        n127 = call-poly "Enqueue Message.vi"("Priority Message? (F)"=TRUE, "error in (no error)"=w336, "Message"="Initialize", "Message Queue"=w337) -> ("error out"=w335:errorcluster)  [unwired: 6 in, 1 out]
        n128 = Merge Errors(w335) -> (w341:errorcluster)
      }
      frame "Set Limits" {
        # "Set the maximum / minimum outputs for this channel"
        n129 = Variant To Data(type=T14 {"Output channel"=enum."1", "Max_Ctrl1"=0.0, "Min_Ctrl1"=0.0} ("output cluster"), Variant=w349) -> (data=w350:T14)  [unwired: 1 in, 1 out]
        n130 = Unbundle By Name(w350) -> ("Max_Ctrl1"=w346:dbl, "Output channel"=w345:T5, "Min_Ctrl1"=w344:dbl)
        n131 = Unbundle By Name(w348) -> ("VISA resource name"=w343:refnum<visa-resource-name>)
        n132 = call "Set-Limits.vi"("Minimum / V"=w344, "Maximum / V"=w346, "Output channel"=w345, "VISA resource name"=w343) -> ("error out"=w342:errorcluster)  [unwired: 2 in, 1 out]
      }
      frame "Get Limits" {
        w351 = T10."Enabled" ("Disabled")
        # "Write new values to their controls"
        # "Decode parameters to output channel"
        # "Get the maximum / minimum outputs for this channel and \nstore them in the appropriate controls"
        n133 = Unbundle By Name(w364) -> ("VISA resource name"=w363:refnum<visa-resource-name>)
        n134 = Variant To Data(type=OutputChannelTypedef."1" ("NewVal"), Variant=w365) -> (data=w354:T5, error out=w362:errorcluster)  [unwired: 1 in]
        n135 = control-ref of="Max_Ctrl"() -> (w353:refnum<vi>)
        n136 = call "Query-Limits.vi"("error in (no error)"=w362, "Output channel"=w354, "VISA resource name"=w363) -> ("error out"=w359:errorcluster, "Recalled minimum / V"=w360:dbl, "Recalled maximum / V"=w361:dbl)  [unwired: 2 in, 1 out]
        n137 = control-ref of="Min_Ctrl"() -> (w352:refnum<vi>)
        n138 = property class="DigNum (strict)"(reference=w352, "Value"=w360, "DisabledEnum"=w351) -> (error out=w357:errorcluster)  [unwired: 1 in, 1 out]
        n139 = property class="DigNum (strict)"(reference=w353, "Value"=w361, "DisabledEnum"=w351) -> (error out=w358:errorcluster)  [unwired: 1 in, 1 out]
        n140 = Merge Errors(w358, w359, w357) -> (w356:errorcluster)
      }
      frame "Get ctrl" {
        # "Write new values to their controls"
        # "Decode parameters to output channel"
        # "Get the current output for this channel and \nstore it in the appropriate control"
        n141 = Unbundle By Name(w376) -> ("VISA resource name"=w370:refnum<visa-resource-name>)
        n142 = Variant To Data(type=OutputChannelTypedef."1" ("NewVal"), Variant=w377) -> (data=w368:T5, error out=w369:errorcluster)  [unwired: 1 in]
        n143 = control-ref of="CtrlVoltage"() -> (w372:refnum<vi>)
        n144 = call "Query-ControlSignal.vi"("error in (no error)"=w369, "Output channel"=w368, "VISA resource name"=w370) -> ("error out"=w367:errorcluster, "Recalled Control signal / V"=w366:dbl)  [unwired: 6 in, 1 out]
        n145 = property class="DigNum (strict)"(reference=w372, "Value"=w366, "DisabledEnum"=T10."Enabled" ("Disabled")) -> (error out=w375:errorcluster)  [unwired: 1 in, 1 out]
        n146 = Merge Errors(w375, w367) -> (w374:errorcluster)
      }
      frame "Start Const Voltage" {
        # "Set a const. voltage output on the given channel"
        n147 = Variant To Data(type=T15 {"Output channel"=enum."1", "Voltage outer"=0.0} ("output cluster"), Variant=w385) -> (data=w382:T15)  [unwired: 1 in, 1 out]
        n148 = Unbundle By Name(w384) -> ("VISA resource name"=w383:refnum<visa-resource-name>)
        n149 = Unbundle By Name(w382) -> ("Output channel"=w380:T5, "Voltage outer"=w379:dbl)
        n150 = call "Set-ConstantOutput.vi"("Voltage / Volts"=w379, "Output channel"=w380, "VISA resource name"=w383) -> ("error out"=w378:errorcluster)  [unwired: 3 in, 1 out]
        n151 = Merge Errors(w378) -> (w386:errorcluster)
      }
      frame "Exit" {
        # "Close text files"
        # "Close the COM port"
        # "Fire the \"Exit\" event to kill the other two loops"
        # "Stop the VI"
        # "Release the message queue reference"
        # "Exit - Exit the application."
        n152 = Unbundle By Name(w393) -> ("VISA resource name"=w392:refnum<visa-resource-name>, "Log file"=w389:refnum<file>)
        n153 = call "Fire User Event - Stop.vi"("User Event - Stop"=w394) -> ("error out"=w391:errorcluster)  [unwired: 10 in]
        n154 = Close File(refnum=w389) -> (error out=w388:errorcluster)  [unwired: 1 in, 1 out]
        n155 = Release Queue(queue=w398, error in (no error)=w395) -> (error out=w387:errorcluster)  [unwired: 1 in, 2 out]
        n156 = call "Close.vi"("VISA resource name"=w392) -> ("error out"=w390:errorcluster)  [unwired: 10 in]
        n157 = Merge Errors(w391, w390, w388, w387) -> (w396:errorcluster)
      }
      frame Default {
        # "'Default' case only runs if there is a message that isn't defined in any of the other cases.  Output a programming error."
        n158 = xnode "Error Ring"("parameter 0"=w399) -> ("error out"=w400:errorcluster)
      }
    }
    n159 = call "Error Handler - Message Handling Loop.vi"("error in (no error)"=w20, "Message Queue"=w22) -> ("dup error in"=w21:errorcluster)  [unwired: 8 in, 1 out]
  }
  n160 = while {
    tunnel: w2 -> [w416]
    tunnel: w4 -> [w415]
    tunnel: [w414] -> w5
    shift-right: [w412] -> _
    shift-left: w1 -> [w413]
    tunnel: w10 -> [w417]
    stop <- w418 stop-if-true
    # "Trigger data logging"
    n161 = Multiply(x=1000, y="Trigger time / s") -> (x*y=w410:i32)
    n162 = event shown="[1] Timeout" {
      selector: w416 -> [_ _ w426]
      dyn-events: _ -> [_ _ _]
      timeout: w410 -> [_ _ _]
      tunnel: [_ _ TRUE] -> w418
      tunnel: w417 -> [_ w422 _]
      tunnel: w415 -> [_ _ w428]
      tunnel: [_ _ w427] -> w414
      tunnel: w413 -> [_ w420 w425]
      tunnel: [TRUE FALSE w425] -> w412
      event User Event {
        # "Mark as ready for data again, starting the timeout timer"
        n163 = event-data() -> ()  [unwired: 1 in, 1 out]
      }
      event Timeout {
        n164 = event-data() -> ()  [unwired: 1 in, 3 out]
        n165 = case shown="False" w420 {
          tunnel: w422 -> [_ w424]
          frame False {
          }
          frame True {
            # "After waiting \"trigger time\" seconds since the last \n\"Logging done\" event, queue data taking"
            n166 = call-poly "Enqueue Message.vi"("Message"="Take data", "Message Queue"=w424) -> ()  [unwired: 8 in, 2 out]
          }
        }
      }
      event User Event {
        # "Unregister for both events, then destroy the  \"Log Data\" user event"
        # "\"Stop\" event triggered: end the loop"
        n167 = event-data() -> ()  [unwired: 1 in, 2 out]
        n168 = Unregister For Events(event registration refnum=w426) -> (error out=w429:errorcluster)  [unwired: 1 in]
        n169 = Destroy User Event(user event=w428, error in=w429) -> (error out=w427:errorcluster)
      }
    }
  }
  n170 = while {
    tunnel: w10 -> [w437]
    shift-right: [w436] -> w14
    shift-left: w9 -> [w431]
    tunnel: [w432] -> w11
    stop <- w434 stop-if-true
    # "Event Handling Loop"
    n171 = event shown="[12] \"Config input channel selector\": Value Change" {
      selector: w431 -> [_ _ _ _ _ _ _ _ _ _ _ _ _ _]
      dyn-events: [_ _ _ _ _ _ _ _ _ _ _ _ _ _] -> w436
      timeout: _ -> [_ _ _ _ _ _ _ _ _ _ _ _ _ _]
      tunnel: [_ _ _ _ _ _ _ _ _ _ _ _ _ TRUE ("Discard?")] -> w434
      tunnel: w437 -> [w448 w454 w460 w473 w483 w486 w497 w509 w513 w518 w520 w525 w529 w531]
      tunnel: [w443 w452 w456 _ _ _ w492 w502 w510 w517 _ w524 _ _] -> w435
      tunnel: [w442 w451 w459 w472 w482 w485 w496 w498 w512 w516 w520 w523 w529 w531] -> w433
      event "Start Lock": Value Change {
        # "Trigger limit setting:"
        # "Start voltage lock"
        n172 = event-data() -> ()  [unwired: 1 in, 1 out]
        n173 = Bundle("Lock settings"="Lock settings", "Output channel"="Output channel", "Input channel"="Input channel") -> (w446:T21)  [unwired: 1 in]
        n174 = call-poly "Enqueue Message.vi"("Message Data"=w446, "Message"="Start Voltage Lock", "Message Queue"=w448) -> ("error out"=w441:errorcluster, "dup Message Queue"=w442:refnum<queue>)  [unwired: 7 in]
        n175 = property on="Max_Ctrl" class="DigNum (strict)"(error in=w441) -> (error out=w444:errorcluster, "Value"=w445:dbl)  [unwired: 1 in, 1 out]
        n176 = property on="Max_Ctrl" class="DigNum (strict)"(error in=w444, "Val(Sgnl)"=w445) -> (error out=w443:errorcluster)  [unwired: 1 in, 1 out]
      }
      event Value Change {
        w455 = T10."Disabled and Grayed Out" ("Disabled")
        # "On \"Output channel\" change, reload the limits for this channel\nAlso, disable related controls until they are refreshed"
        n177 = event-data() -> ("NewVal"=w449:T5)  [unwired: 1 in, 2 out]
        n178 = Build Array(w449, w449) -> (w450:T5[])
        n179 = call-poly "Enqueue Message.vi"("Message Data Array"=w450, "Message Array"=string[] ["Get limits", "Get ctrl"], "Message Queue"=w454) -> ("error out"=w452:errorcluster, "dup Message Queue"=w451:refnum<queue>)  [unwired: 7 in]
        n180 = property on="Max_Ctrl" class="DigNum (strict)"("DisabledEnum"=w455) -> ()  [unwired: 2 in, 2 out]
        n181 = property on="Min_Ctrl" class="DigNum (strict)"("DisabledEnum"=w455) -> ()  [unwired: 2 in, 2 out]
        n182 = property on="CtrlVoltage" class="DigNum (strict)"("DisabledEnum"=w455) -> ()  [unwired: 2 in, 2 out]
      }
      event "Log file prefix": Value Change {
        # "If the enable logging switch is switched, stop and restart logging with the new filename"
        n183 = event-data() -> ()  [unwired: 1 in, 2 out]
        n184 = property on="Enable logging" class="Bool (strict)"() -> (error out=w457:errorcluster, "Value"=w458:bool)  [unwired: 2 in, 1 out]
        n185 = case shown="True" w458 {
          tunnel: w460 -> [w462 w470]
          tunnel: [w462 w466] -> w459
          tunnel: w457 -> [w461 w465]
          tunnel: [w461 w463] -> w456
          frame False {
          }
          frame True {
            n186 = call-poly "Enqueue Message.vi"("error in (no error)"=w465, "Message"="Stop logging", "Message Queue"=w470) -> ("error out"=w464:errorcluster, "dup Message Queue"=w467:refnum<queue>)  [unwired: 7 in]
            n187 = call-poly "Enqueue Message.vi"("error in (no error)"=w464, "Message"="Start logging", "Message Queue"=w467) -> ("error out"=w463:errorcluster, "dup Message Queue"=w466:refnum<queue>)  [unwired: 7 in]
          }
        }
      }
      event "Enable logging": Value Change {
        n188 = event-data() -> ()  [unwired: 1 in, 2 out]
        n189 = case shown="False" "Enable logging" {
          tunnel: w473 -> [w476 w479]
          tunnel: [w474 w477] -> w472
          frame True {
            n190 = call-poly "Enqueue Message.vi"("Message"="Start logging", "Message Queue"=w476) -> ("dup Message Queue"=w474:refnum<queue>)  [unwired: 8 in, 1 out]
          }
          frame False {
            n191 = call-poly "Enqueue Message.vi"("Message"="Stop logging", "Message Queue"=w479) -> ("dup Message Queue"=w477:refnum<queue>)  [unwired: 8 in, 1 out]
          }
        }
      }
      event "Error abort": Value Change {
        # "Abort the software in response to an error"
        n192 = event-data() -> ()  [unwired: 1 in, 2 out]
        n193 = call-poly "Enqueue Message.vi"("Priority Message? Array"=bool[] [TRUE, TRUE], "Message Array"=string[] ["Hide error bar", "Exit"], "Message Queue"=w483) -> ("dup Message Queue"=w482:refnum<queue>)  [unwired: 7 in, 1 out]
      }
      event "Error ignore": Value Change {
        # "Abort the software in response to an error"
        n194 = event-data() -> ()  [unwired: 1 in, 2 out]
        n195 = call-poly "Enqueue Message.vi"("Message"="Hide error bar", "Message Queue"=w486) -> ("dup Message Queue"=w485:refnum<queue>)  [unwired: 8 in, 1 out]
      }
      event "Start Const.Voltage": Value Change {
        # "Trigger set limits event"
        # "Const. Voltage"
        n196 = event-data() -> ()  [unwired: 1 in, 2 out]
        n197 = property on="Output channel" class="Enum (strict)"() -> ("Value"=w488:T5)  [unwired: 2 in, 2 out]
        n198 = Bundle By Name(cluster=T15 {"Output channel"=enum."1", "Voltage outer"=0.0} ("output cluster"), "Output channel"=w488, "Voltage outer"="CtrlVoltage") -> (w494:T15)
        n199 = call-poly "Enqueue Message.vi"("Message Data"=w494, "Message"="Start Const Voltage", "Message Queue"=w497) -> ("error out"=w490:errorcluster, "dup Message Queue"=w496:refnum<queue>)  [unwired: 7 in]
        n200 = property on="Max_Ctrl" class="DigNum (strict)"(error in=w490) -> (error out=w491:errorcluster, "Value"=w489:dbl)  [unwired: 1 in, 1 out]
        n201 = property on="Max_Ctrl" class="DigNum (strict)"(error in=w491, "Val(Sgnl)"=w489) -> (error out=w492:errorcluster)  [unwired: 1 in, 1 out]
      }
      event "Max_Ctrl", "Min_Ctrl": Value Change {
        # "Set output channel limits (then get them to check it went through ok)"
        n202 = event-data() -> ()  [unwired: 1 in, 2 out]
        n203 = property on="Output channel" class="Enum (strict)"() -> ("Value"=w500:T5)  [unwired: 2 in, 2 out]
        n204 = Bundle By Name(cluster=T14 {"Output channel"=enum."1", "Max_Ctrl1"=0.0, "Min_Ctrl1"=0.0} ("output cluster"), "Output channel"=w500, "Max_Ctrl1"="Max_Ctrl", "Min_Ctrl1"="Min_Ctrl") -> (w505:T14)
        n205 = call-poly "Enqueue Message.vi"("Message Data"=w505, "Message"="Set limits", "Message Queue"=w509) -> ("error out"=w501:errorcluster, "dup Message Queue"=w499:refnum<queue>)  [unwired: 7 in]
        n206 = call-poly "Enqueue Message.vi"("error in (no error)"=w501, "Message Data"=w500, "Message"="Get limits", "Message Queue"=w499) -> ("error out"=w502:errorcluster, "dup Message Queue"=w498:refnum<queue>)  [unwired: 6 in]
      }
      event "Reset": Value Change {
        # "Reset the device"
        n207 = event-data() -> ()  [unwired: 1 in, 1 out]
        n208 = call-poly "Enqueue Message.vi"("Message"="Reset", "Message Queue"=w513) -> ("error out"=w510:errorcluster, "dup Message Queue"=w512:refnum<queue>)  [unwired: 8 in]
      }
      event Panel Close? {
        # "Send the 'Confirm Quit' message if the user closes the panel of the VI. Discard the event so the 'Confirm Quit' message has a chance to run."
        n209 = event-data() -> ()  [unwired: 1 in, 1 out]
        n210 = call-poly "Enqueue Message.vi"("Priority Message? (F)"=TRUE, "Message"="Confirm Quit", "Message Queue"=w518) -> ("error out"=w517:errorcluster, "dup Message Queue"=w516:refnum<queue>)  [unwired: 7 in]
        n211 = event-data("Discard?"=TRUE) -> ()  [unwired: 1 in, 1 out]
      }
      event Application Instance Close {
        # "#CodeRecommended - When a project closes, all VIs within that project are aborted and leave memory. However, any code placed in this event frame is guaranteed to run to completion, so add any cleanup code that absolutely must happen here."
        n212 = event-data() -> ()  [unwired: 1 in, 1 out]
      }
      event "Exit": Value Change {
        n213 = event-data() -> ()  [unwired: 1 in, 1 out]
        n214 = call-poly "Enqueue Message.vi"("Priority Message? Array"=bool[] [TRUE, TRUE], "Message Array"=string[] ["Hide error bar", "Exit"], "Message Queue"=w525) -> ("error out"=w524:errorcluster, "dup Message Queue"=w523:refnum<queue>)  [unwired: 7 in]
      }
      event Value Change {
        # "Update the thermistor config array to show the right value\nwhen the selector is changed"
        n215 = event-data() -> ()  [unwired: 1 in, 2 out]
        n216 = To Unsigned Long Integer(number="Config input channel selector") -> (unsigned 32bit integer=w526:u32)
        n217 = Build Array(w526) -> (w528:u32[])
        n218 = property on="Input arm settings" class="Arr (strict)"("Index Values"=w528) -> ()  [unwired: 2 in, 2 out]
      }
      event User Event {
        # "The Message Handling Loop processed an \"Exit\" message, which fired this event to stop the Event Handling Loop."
        n219 = event-data() -> ()  [unwired: 1 in, 4 out]
      }
    }
    n220 = call "Error Handler - Event Handling Loop.vi"("error in (no error)"=w435, "Message Queue"=w433) -> ("dup error in"=w432:errorcluster)  [unwired: 8 in, 1 out]
  }
  n221 = Merge Errors(w11, w7, w5) -> (w12:errorcluster)
  n222 = Unregister For Events(event registration refnum=w14, error in=w12) -> (error out=w6:errorcluster)
  n223 = call "Destroy User Event - Stop.vi"("error in (no error)"=w6, "User Event - Stop"=w3) -> ()  [unwired: 9 in, 1 out]
